vi "API_DB.UpdateRecord.vi"(6 "Timeout (ms)":u32, 7 "Wait (F)":bool, 8 "error in (no error)":errorcluster, 10 "QueryBuilderData":T1, 11 "Database in":refnum<class "Database.lvclass">) -> (0 "error out":errorcluster, 3 "Database out":refnum<class "Database.lvclass">)   [LabVIEW 2022 SP3, in "Database.lvclass"]
doc: "Developed by Kevin Thompson\nkevin@thompsonengineering.net\n\nCopyright 2018\nThompson Engineering, LLC"
uses:
  Database.lvclass
  DataTypes/QuiryBuilderData--Cluster.ctl
  DataTypes/AsynCmd_Temp01--enum.ctl
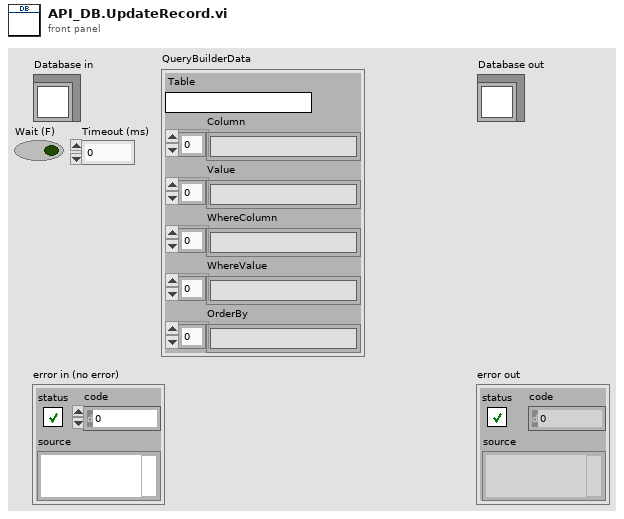
[diagram p1: front panel]
types:
  T1 = typedef "QuiryBuilderData--Cluster.ctl" = cluster{"Table":string, "Column":string[], "Value":string[], "WhereColumn":string[], "WhereValue":string[], "OrderBy":string[]}
  T2 = typedef "Database.lvclass/AsynCmd_Temp01--enum.ctl" = enum16{"DB.DeleteRecord", "DB.UpdateRecord", "DB.InsertRecord", "DB.SelectRecord", "DB.ExecuteSQLCommand", "DB.FindFirstSlot", "DB.GenericSQLQuery"}
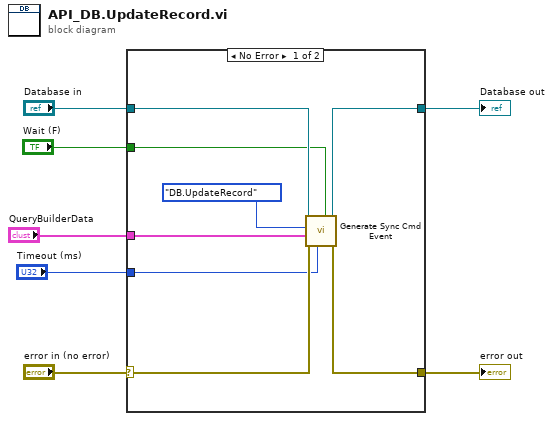
[diagram p0: block diagram]
diagram:
  n1 = case shown="No Error" "error in (no error)" {
    selector: "error in (no error)" -> [w13 w17]
    tunnel: [w12 w17] -> w6
    tunnel: [w14 w16] -> w4
    tunnel: "Database in" -> [w15 w16]
    tunnel: "QueryBuilderData" -> [w10 _]
    tunnel: "Wait (F)" -> [w9 _]
    tunnel: "Timeout (ms)" -> [w8 _]
    frame No Error {
      n2 = call "Generate Sync Cmd Event.vi"("Wait (F)"=w9, "Timeout (ms)"=w8, "error in (no error)"=w13, "vData"=w10, "AsyncCmd"=AsynCmd_Temp01--enum."DB.UpdateRecord", "Database in"=w15) -> ("error out"=w12:errorcluster, "Database out"=w14:refnum<class "Database.lvclass">)  [unwired: 3 in, 1 out]
    }
    frame Error {
    }
  }
  "error out" <- w6
  "Database out" <- w4
